vi "Packet Encode.vi"(8 "error in (no error)":errorcluster, 11 "Map in":refnum<class "Map.lvclass">) -> (0 "error out":errorcluster, 2 "Data":u8[](array[numeric]), 3 "Map out":refnum<class "Map.lvclass">)   [LabVIEW 2019, in "Map.lvclass"]
uses:
  Map.lvclass
  TCP Packet/Packet.lvclass
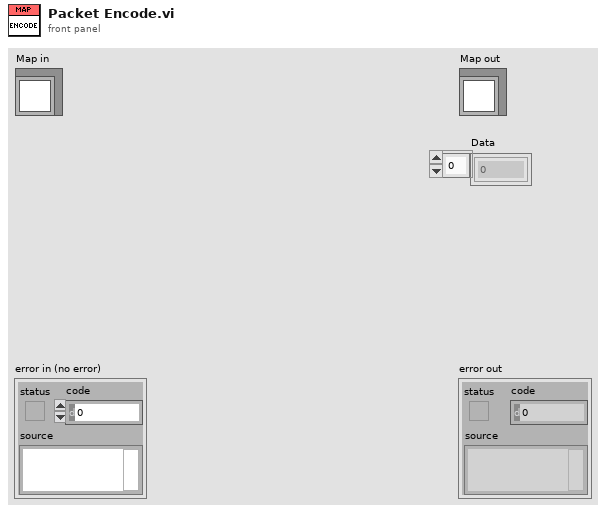
[diagram p1: front panel]
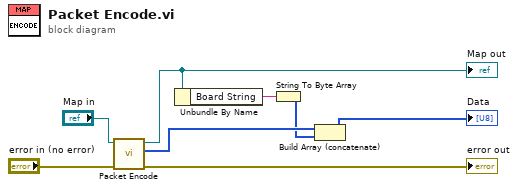
[diagram p0: block diagram]
diagram:
  n1 = call-parent "Packet Encode.vi"("error in (no error)"="error in (no error)", "Packet in"="Map in") -> ("error out"=→"error out":errorcluster, "Data"=w3:u8[], "Packet out"=w5:refnum<class "Map.lvclass">)  [unwired: 7 in]
  "Map out" <- w5
  n2 = Unbundle By Name(w5) -> ("Board String"=w4:string)
  n3 = String To Byte Array(string=w4) -> (unsigned byte array=w2:u8[])
  n4 = Build Array (concatenate)(w3, w2) -> (→"Data":u8[])
